vi "type.vi"(8 "Error In":errorcluster, 11 "QWindow In":refnum<class "QWindow.lvclass">) -> (0 "Error Out":errorcluster, 2 "Value":T1 items=["Widget"=0, "Window"=1, "Dialog"=3, "Sheet"=5, "Drawer"=7, "Popup"=9, "Tool"=11, "ToolTip"=13, "SplashScreen"=15, "Desktop"=17, "SubWindow"=18, "ForeignWindow"=33, "CoverWindow"=65, "WindowType_Mask"=255, "MSWindowsFixedSizeDialogHint"=256, "MSWindowsOwnDC"=512, "BypassWindowManagerHint"=1024, "FramelessWindowHint"=2048, "WindowTitleHint"=4096, "WindowSystemMenuHint"=8192, "WindowMinimizeButtonHint"=16384, "WindowMaximizeButtonHint"=32768, "WindowMinMaxButtonsHint"=49152, "WindowContextHelpButtonHint"=65536, "WindowShadeButtonHint"=131072, "WindowStaysOnTopHint"=262144, "WindowTransparentForInput"=524288, "WindowOverridesSystemGestures"=1048576, "WindowDoesNotAcceptFocus"=2097152, "CustomizeWindowHint"=33554432, "WindowStaysOnBottomHint"=67108864, "WindowCloseButtonHint"=134217728, "MacWindowToolBarButtonHint"=268435456, "BypassGraphicsProxyWidget"=536870912, "NoDropShadowWindowHint"=1073741824, "WindowFullscreenButtonHint"=-2147483648], 3 "QWindow Out":refnum<class "QWindow.lvclass">)   [LabVIEW 2014, in "QWindow.lvclass"]
doc: "LabVIEW-specific documentation is not yet available. See <b>http://doc.qt.io/qt-5/QWindow.html#type</b>"
uses:
  QWindow.lvclass
  LQ Core/Qt/WindowType.ctl
  LQ Core/LQIdentity/LQIdentity.lvclass/LQIdentity.ctl
  LQ Core/LQ Core.lvlib
  LQ Core/LQIdentity/LQIdentity.lvclass
  LQ Core/Qt/Qt.lvlib
panel:
  # "Copyright (c) 2016 Sze Howe Koh\n\nThis Source Code Form is subject to the terms of the Mozilla Public\nLicense, v. 2.0. If a copy of the MPL was not distributed with this\nfile, You can obtain one at http://mozilla.org/MPL/2.0/."
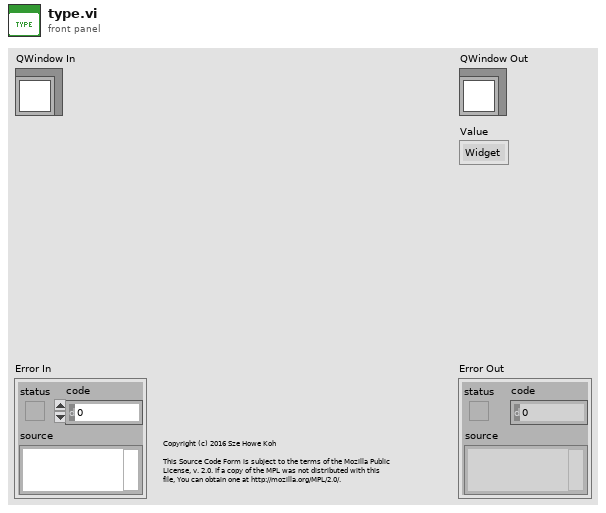
[diagram p1: front panel]
types:
  T1 = typedef "Qt.lvlib/WindowType.ctl" = i32
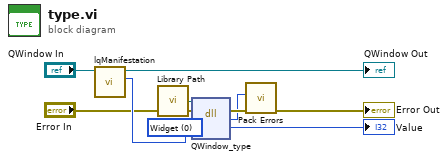
[diagram p0: block diagram]
diagram:
  w7 = T1 0 items=["Widget"=0, "Window"=1, "Dialog"=3, "Sheet"=5, "Drawer"=7, "Popup"=9, "Tool"=11, "ToolTip"=13, "SplashScreen"=15, "Desktop"=17, "SubWindow"=18, "ForeignWindow"=33, "CoverWindow"=65, "WindowType_Mask"=255, "MSWindowsFixedSizeDialogHint"=256, "MSWindowsOwnDC"=512, "BypassWindowManagerHint"=1024, "FramelessWindowHint"=2048, "WindowTitleHint"=4096, "WindowSystemMenuHint"=8192, "WindowMinimizeButtonHint"=16384, "WindowMaximizeButtonHint"=32768, "WindowMinMaxButtonsHint"=49152, "WindowContextHelpButtonHint"=65536, "WindowShadeButtonHint"=131072, "WindowStaysOnTopHint"=262144, "WindowTransparentForInput"=524288, "WindowOverridesSystemGestures"=1048576, "WindowDoesNotAcceptFocus"=2097152, "CustomizeWindowHint"=33554432, "WindowStaysOnBottomHint"=67108864, "WindowCloseButtonHint"=134217728, "MacWindowToolBarButtonHint"=268435456, "BypassGraphicsProxyWidget"=536870912, "NoDropShadowWindowHint"=1073741824, "WindowFullscreenButtonHint"=-2147483648] ("retVal")
  n1 = call "lqManifestation.vi"("LQIdentity in"="QWindow In") -> ("Manifestation"=w5:u64, "LQIdentity out"=→"QWindow Out":refnum<class "QWindow.lvclass">)  [unwired: 9 in]
  n2 = call "Library Path.vi"() -> ("Library Path"=w6:path)
  n3 = dll-call lib="?" fn="QWindow_type"(path in=w6, error in="Error In", "_retVal"=w7, "_instance"=w5) -> (error out=w3:errorcluster, w1:i32, "_retVal"=→"Value":i32)  [unwired: 2 in, 1 out]
  n4 = call "Pack Errors.vi"("Error In"=w3, "Error Code"=w1) -> ("Error Out"=→"Error Out":errorcluster)  [unwired: 9 in]
